vi "AMC Send Local Messages.vi"(4 "Message Attributes":T1[](array[typedef]), 7 "Process (\"\" - local)":string, 8 "error in (no error)":errorcluster, 9 "Message Values":string[](array[string]), 10 "Message Names":string[](array[string]), 11 "Message Queue in":T2) -> (0 "error out":errorcluster, 3 "Message Queue out":T2)   [LabVIEW 2012, in "REx_Springboard.lvlib" / "TLB_Dependencies.lvlib"]
doc: "This VI adds one or more messages to the local message queue provided by the queue reference or to another message queue on the local target based on the receiver process name."
uses:
  TLB_Dependencies.lvlib
  amc_Message Queue.ctl
  amc_Message.ctl
  <vilib>/FTP/util/Keyed Array.ctl
  <vilib>/FTP/NI_FTP.lvlib
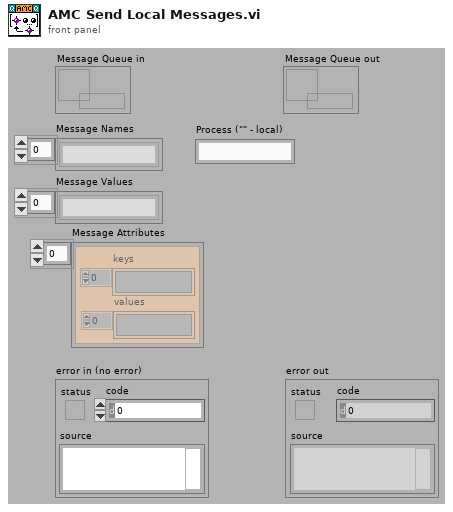
[diagram p1: front panel]
types:
  T1 = typedef "NI_FTP.lvlib/Keyed Array.ctl" = cluster{"keys":string[], "values":string[]}
  T2 = typedef "REx_Springboard.lvlib/TLB_Dependencies.lvlib/amc_Message Queue.ctl" = refnum<queue>
  T3 = typedef "REx_Springboard.lvlib/TLB_Dependencies.lvlib/amc_Message.ctl" = cluster{"Name":string, "Value":string, "Attributes":T1, "Receiver Host":string, "Receiver Process":string, "Source Host":string, "Source Process":string, "Priority Message":bool, "Acknowledge Message":bool}
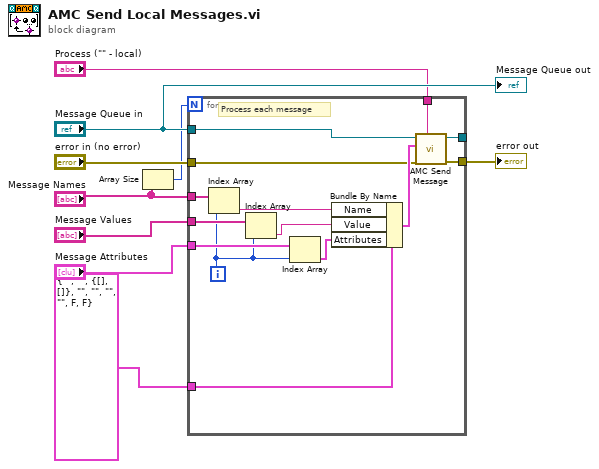
[diagram p0: block diagram]
diagram:
  n1 = Array Size(array="Message Names") -> (size(s)=w3:i32)
  n2 = for {
    N: w3 -> [_]
    tunnel: "Message Queue in" -> [w22]
    tunnel: [w21] -> _
    tunnel: "error in (no error)" -> [w20]
    tunnel: [w19] -> w8
    tunnel: "Message Values" -> [w18]
    tunnel: "Message Names" -> [w17]
    tunnel: "Message Attributes" -> [w16]
    tunnel: "Process (\"\" - local)" -> [w11]
    tunnel: T3 {"Name"="", "Value"="", "Attributes"={"keys"=[], "values"=[]}, "Receiver Host"="", "Receiver Process"="", "Source Host"="", "Source Process"="", "Priority Message"=FALSE, "Acknowledge Message"=FALSE} ("Message") -> [w10]
    i -> [w12]
    # "Process each message"
    n3 = Index Array(array=w17, index=w12) -> (element=w15:string)
    n4 = Index Array(array=w18, index=w12) -> (element=w14:string)
    n5 = Index Array(array=w16, index=w12) -> (element=w13:T1)
    n6 = Bundle By Name(cluster=w10, "Name"=w15, "Value"=w14, "Attributes"=w13) -> (w23:T3)
    n7 = call "AMC Send Message.vi"("Receiver Process"=w11, "error in (no error)"=w20, "Message"=w23, "Message Queue in"=w22) -> ("error out"=w19:errorcluster, "Message Queue out"=w21:T2)  [unwired: 4 in, 2 out]
  }
  "error out" <- w8
  "Message Queue out" <- "Message Queue in"
